vi "peakRef.vi"(8 "error in (no error)":errorcluster, 11 "Prueba09 in":refnum<class "Prueba09.lvclass">) -> (0 "error out":errorcluster, 2 "tablaPeakRef[dB]":string[](array[string]), 3 "Prueba09 out":refnum<class "Prueba09.lvclass">)   [LabVIEW 2019, in "Prueba09.lvclass"]
uses:
  Prueba09.lvclass
  Prueba09.lvclass/Prueba09.ctl
  Prueba/Prueba.lvclass
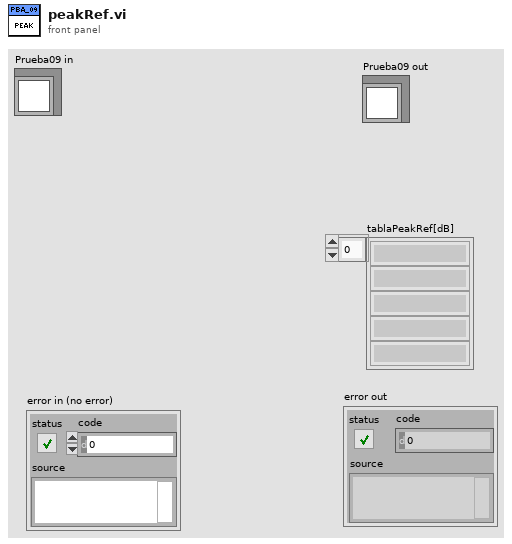
[diagram p1: front panel]
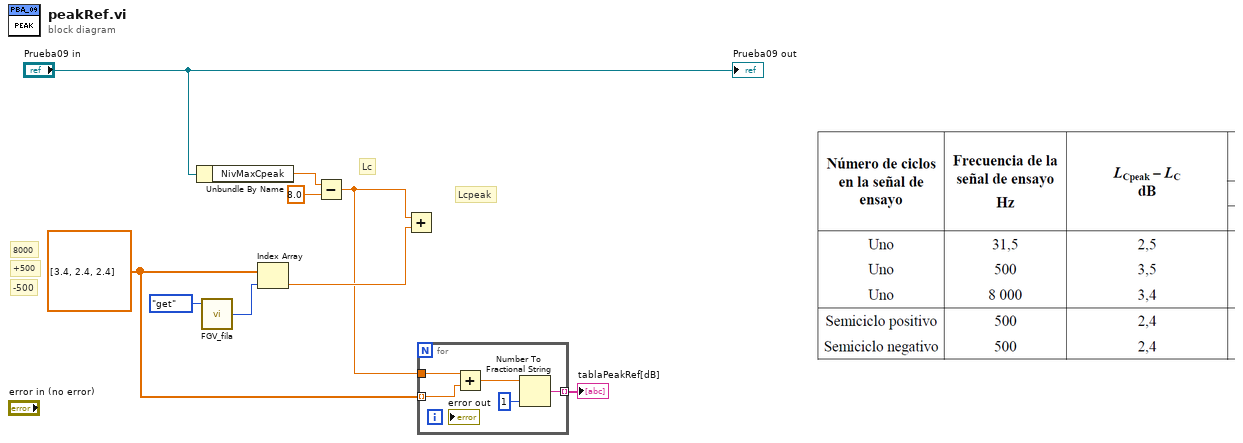
[diagram p0: block diagram]
diagram:
  w4 = dbl[] [3.4, 2.4, 2.4]
  # "Lcpeak"
  # "Lc"
  # "-500"
  # "+500"
  # "8000"
  n1 = Unbundle By Name("Prueba09 in") -> ("NivMaxCpeak"=w9:dbl)
  n2 = call "FGV_fila.vi"("action"=enum16{"increment", "set_start", "get"}."get") -> ("fila out"=w6:i32)  [unwired: 3 in, 1 out]
  n3 = Index Array(array=w4, index=w6) -> (element=w5:dbl)
  n4 = Subtract(x=w9, y=8.0) -> (x-y=w3:dbl)
  n5 = Add(x=w3, y=w5) -> ()  [unwired: 1 out]
  n6 = for {
    tunnel: w4 -> [w13] mode=indexing
    tunnel: w3 -> [w14]
    tunnel: [w10] -> w2 mode=indexing
    n7 = Add(x=w14, y=w13) -> (x+y=w11:dbl)
    n8 = Number To Fractional String(number=w11, precision (6)=i16 1) -> (F-format string=w10:string)  [unwired: 2 in]
  }
  "tablaPeakRef[dB]" <- w2
  "Prueba09 out" <- "Prueba09 in"
